vi "3020仪器参数发送.vi"   [LabVIEW 2016, in "数据传输系统.lvlib"]
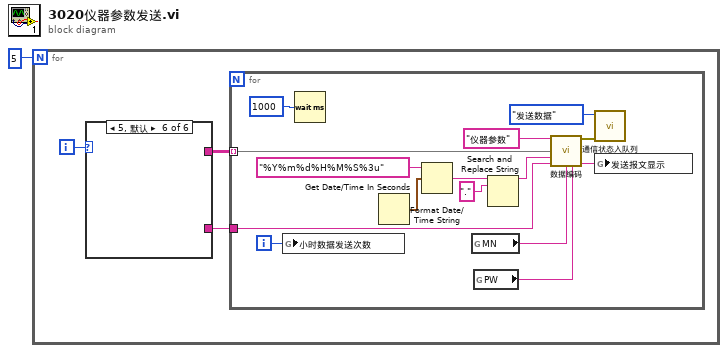
[diagram p0: block diagram]
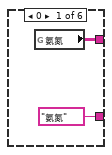
[diagram p2: hidden frame]
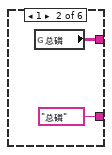
[diagram p3: hidden frame]
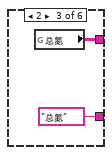
[diagram p4: hidden frame]
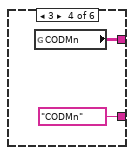
[diagram p5: hidden frame]
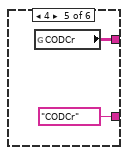
[diagram p6: hidden frame]
diagram:
  n1 = for {
    N: 5 -> [_]
    i -> [w4]
    n2 = case shown="5, 默认" w4 {
      tunnel: [w6 w8 w10 w12 w14 _] -> w3
      tunnel: ["氨氮" ("污染物编码") "总磷" ("污染物编码") "总氮" ("污染物编码") "CODMn" ("污染物编码") "CODCr" ("污染物编码") _] -> w2
      frame 0 {
        n3 = global read "全局 所有参数.vi" "氨氮"() -> (w6:string[][])
      }
      frame 1 {
        n4 = global read "全局 所有参数.vi" "总磷"() -> (w8:string[][])
      }
      frame 2 {
        n5 = global read "全局 所有参数.vi" "总氮"() -> (w10:string[][])
      }
      frame 3 {
        n6 = global read "全局 所有参数.vi" "CODMn"() -> (w12:string[][])
      }
      frame 4 {
        n7 = global read "全局 所有参数.vi" "CODCr"() -> (w14:string[][])
      }
      frame 5, Default {
      }
    }
    n8 = for {
      tunnel: w2 -> [w18]
      tunnel: w3 -> [w17] mode=indexing
      i -> [w16]
      n9 = global write "全局 小时数据发送次数.vi" "小时数据发送次数"(w16) -> ()
      n10 = Wait (ms)(milliseconds to wait=u32 1000 ("等待时间（毫秒）")) -> ()  [unwired: 1 out]
      n11 = Get Date/Time In Seconds() -> (seconds since 1Jan1904=w27:timestamp)
      n12 = Format Date/Time String(time format string (%c)="%Y%m%d%H%M%S%3u" ("时间格式字符串(%c)"), seconds (now)=w27) -> (date/time string=w26:string)  [unwired: 1 in]
      n13 = global read "断电保存全局.vi" "MN"() -> (w21:string)
      n14 = global read "断电保存全局.vi" "PW"() -> (w20:string)
      n15 = Search and Replace String(input string=w26, search string="." ("搜索字符串")) -> (result string=w24:string)  [unwired: 6 in, 3 out]
      n16 = call "数据编码.vi"("table输入"="仪器参数" ("新元素/子数组"), "仪器参数"=w17, "QN"=w24, "参数"=w18, "MN"=w21, "PW"=w20) -> ("错误常量"=w19:errorcluster, "通讯包字符串"=w23:string)  [unwired: 8 in]
      n17 = call "通信状态入队列.vi"("错误输入（无错误）"=w19, "枚举"=enum16{"打开连接", "发送数据", "读取数据", "数据处理", "关闭连接"}."发送数据") -> ()  [unwired: 9 in, 1 out]
      n18 = global write "全局1.vi" "发送报文显示"(w23) -> ()
    }
  }
